vi "Sizeof 1D.vi"(10 "count":u64, 11 "data type":T1) -> (3 "size in bytes":u64 format="%d bytes")   [LabVIEW 2017, in "DSF Core.lvlib"]
uses:
  DSF Core.lvlib
  Configuration/Public/Controls/DSF Data Type.ctl
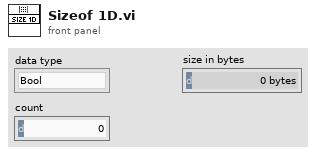
[diagram p1: front panel]
types:
  T1 = typedef "DSF Core.lvlib/DSF Data Type.ctl" = enum8{"Bool", "SGL", "DBL", "I8", "I16", "I32", "I64", "U8", "U16", "U32", "U64"}
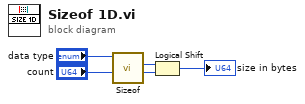
[diagram p0: block diagram]
diagram:
  n1 = call "Sizeof.vi"("data type"="data type") -> ("bitshift count"=w3:u8)  [unwired: 9 in, 1 out]
  n2 = Logical Shift(y=w3, x="count") -> (x << y=→"size in bytes":u64)
